vi "Move relative.vi"(8 "error in (no error)":errorcluster, 10 "Move array":dbl[](array[numeric]), 11 "ConfocalStage in":refnum<class "ConfocalStage.lvclass">) -> (0 "error out":errorcluster, 3 "ConfocalStage out":refnum<class "ConfocalStage.lvclass">)   [LabVIEW 2012, in "ConfocalStage.lvclass"]
uses:
  ConfocalStage.lvclass
  ConfocalStage.lvclass/ConfocalStage.ctl
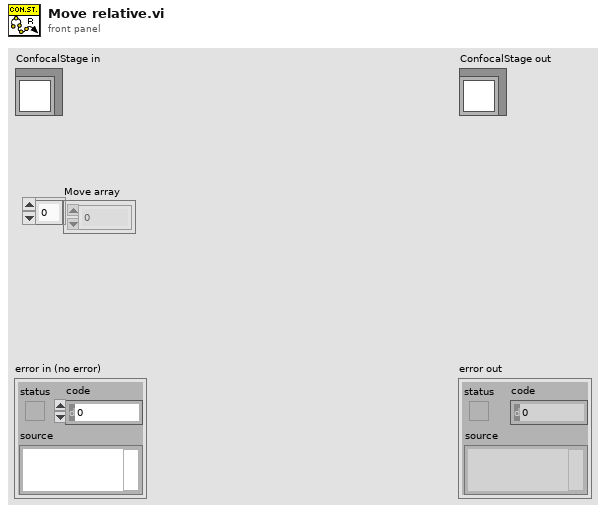
[diagram p1: front panel]
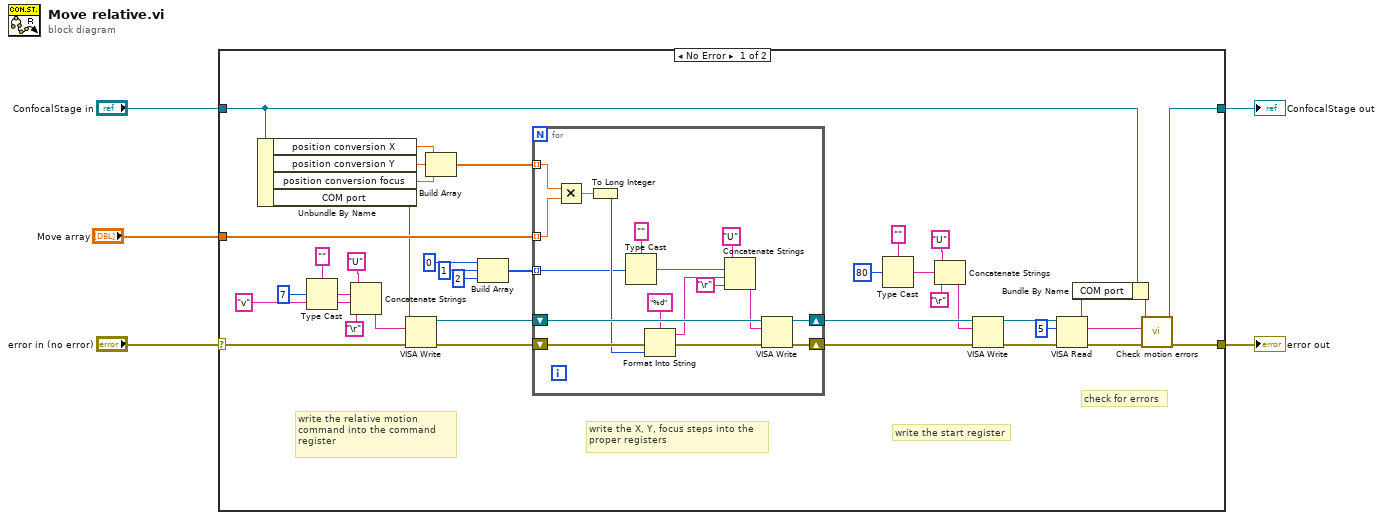
[diagram p0: block diagram]
diagram:
  n1 = case shown="No Error" "error in (no error)" {
    selector: "error in (no error)" -> [w32 w62]
    tunnel: [w13 w62] -> w4
    tunnel: [w11 w61] -> w2
    tunnel: "ConfocalStage in" -> [w12 w61]
    tunnel: "Move array" -> [w43 _]
    frame No Error {
      # "check for errors"
      # "write the start register"
      # "write the X, Y, focus steps into the\nproper registers"
      # "write the relative motion\ncommand into the command\nregister"
      n2 = Unbundle By Name(w12) -> ("position conversion X"=w42:dbl, "position conversion Y"=w41:dbl, "position conversion focus"=w40:dbl, "COM port"=w31:refnum<visa-resource-name>)
      n3 = Type Cast(type="", x=u8 7) -> (*(type *) &x=w37:string)
      n4 = Concatenate Strings("U", w37, "v", "\r") -> (w30:string)
      n5 = VISA Write(VISA resource name=w31, write buffer=w30, error in (no error)=w32) -> (VISA resource name out=w28:refnum<visa-resource-name>, error out=w29:errorcluster)  [unwired: 1 out]
      n6 = Build Array(w42, w41, w40) -> (w39:dbl[])
      n7 = Build Array(u8 0, u8 1, u8 2) -> (w24:u8[])
      n8 = for {
        tunnel: w43 -> [w60] mode=indexing
        tunnel: w39 -> [w59] mode=indexing
        shift-right: [w57] -> w22
        shift-left: w29 -> [w52]
        shift-right: [w45] -> w23
        shift-left: w28 -> [w56]
        tunnel: w24 -> [w47] mode=indexing
        n9 = Multiply(x=w59, y=w60) -> (x*y=w58:dbl)
        n10 = To Long Integer(number=w58) -> (32bit integer=w50:i32)
        n11 = Type Cast(type="", x=w47) -> (*(type *) &x=w54:string)
        n12 = Format Into String(format string="%d", error in=w52, w50) -> (resulting string=w48:string, error out=w51:errorcluster)  [unwired: 1 in]
        n13 = Concatenate Strings("U", w54, w48, "\r") -> (w46:string)
        n14 = VISA Write(VISA resource name=w56, write buffer=w46, error in (no error)=w51) -> (VISA resource name out=w45:refnum<visa-resource-name>, error out=w57:errorcluster)  [unwired: 1 out]
      }
      n15 = Type Cast(type="", x=u8 80) -> (*(type *) &x=w20:string)
      n16 = Concatenate Strings("U", w20, "\r") -> (w17:string)
      n17 = VISA Write(VISA resource name=w23, write buffer=w17, error in (no error)=w22) -> (VISA resource name out=w16:refnum<visa-resource-name>, error out=w33:errorcluster)  [unwired: 1 out]
      n18 = VISA Read(VISA resource name=w16, byte count=u32 5, error in (no error)=w33) -> (VISA resource name out=w9:refnum<visa-resource-name>, read buffer=w15:string, error out=w14:errorcluster)  [unwired: 1 out]
      n19 = Bundle By Name(cluster=w12, "COM port"=w9) -> (w10:refnum<class "ConfocalStage.lvclass">)
      n20 = call-dynamic "Check motion errors.vi"("error in (no error)"=w14, "VISA output string"=w15, "ConfocalStage in"=w10) -> ("error out"=w13:errorcluster, "ConfocalStage out"=w11:refnum<class "ConfocalStage.lvclass">)  [unwired: 7 in]
    }
    frame Error {
    }
  }
  "error out" <- w4
  "ConfocalStage out" <- w2
